vi "Configure Data Format.vi"(0 "VISA resource name":refnum<visa-resource-name>, 5 "Data Format (0:ASCII)":u16(ring) items=["ASCII", "Single Precision (32 bit)"], 9 "Byte Order (1: Normal)":u16(ring)=1 items=["Swapped", "Normal"], 11 "error in (no error)":errorcluster) -> (4 "VISA resource name out":refnum<visa-resource-name>, 15 "error out":errorcluster)   [LabVIEW 2020, in "Keithley 27XX.lvlib"]
doc: "This VI controls how the data is returned and what data is returned from the instrument.\n\nThis VI should not be run with the Model 2701 because it does not support binary transfers."
uses:
  <instrlib>/Keithley 27XX/Keithley 27XX.lvlib
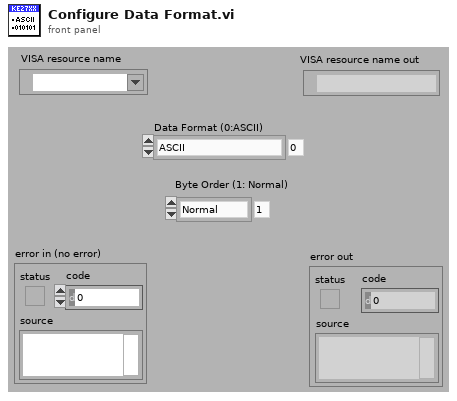
[diagram p1: front panel]
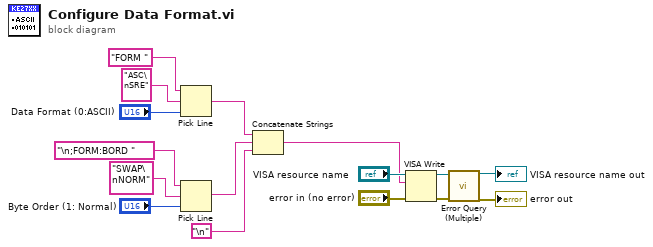
[diagram p0: block diagram]
diagram:
  n1 = Pick Line(string ("")="FORM " ("false string"), multi-line string="ASC\nSRE", line index="Data Format (0:ASCII)") -> (output string=w11:string)
  n2 = Pick Line(string ("")="\n;FORM:BORD ", multi-line string="SWAP\nNORM" ("true string"), line index="Byte Order (1: Normal)") -> (output string=w2:string)
  n3 = Concatenate Strings(w11, w2, "\n") -> (w10:string)
  n4 = VISA Write(VISA resource name="VISA resource name", write buffer=w10, error in (no error)="error in (no error)") -> (VISA resource name out=w9:refnum<visa-resource-name>, error out=w8:errorcluster)  [unwired: 1 out]
  n5 = call <instrlib>:"Error Query (Multiple).vi"("VISA resource name"=w9, "error in (no error)"=w8) -> ("VISA resource name out"=→"VISA resource name out":refnum<visa-resource-name>, "error out"=→"error out":errorcluster)  [unwired: 10 in, 2 out]
